vi "Correlation.vi"(9 "Y":dbl[](array[numeric]), 10 "X":dbl[](array[numeric])) -> (2 "c":dbl)   [LabVIEW 2013]
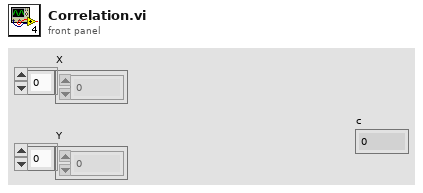
[diagram p1: front panel]
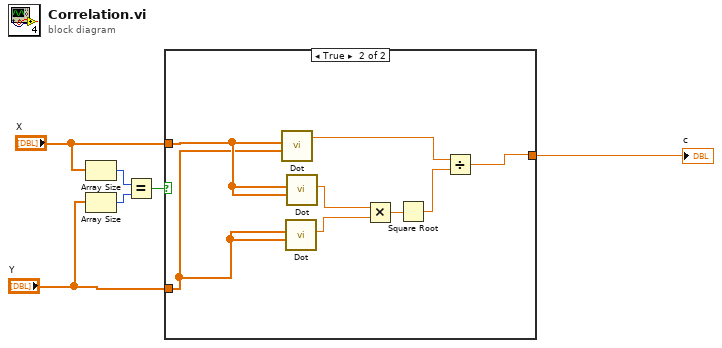
[diagram p0: block diagram]
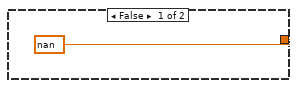
[diagram p2: hidden frame]
diagram:
  n1 = Array Size(array="X") -> (size(s)=w4:i32)
  n2 = Array Size(array="Y") -> (size(s)=w2:i32)
  n3 = Equal?(x=w4, y=w2) -> (x = y?=w5:bool)
  n4 = case shown="True" w5 {
    tunnel: "X" -> [_ w13]
    tunnel: [nan w15] -> w6
    tunnel: "Y" -> [_ w12]
    frame False {
    }
    frame True {
      n5 = call "Dot.vi"("Points Ajustés"=w12, "Y"=w13) -> ("dot(X,Y)"=w14:dbl)  [unwired: 9 in]
      n6 = call "Dot.vi"("Points Ajustés"=w12, "Y"=w12) -> ("dot(X,Y)"=w10:dbl)  [unwired: 9 in]
      n7 = call "Dot.vi"("Points Ajustés"=w13, "Y"=w13) -> ("dot(X,Y)"=w11:dbl)  [unwired: 9 in]
      n8 = Multiply(x=w11, y=w10) -> (x*y=w9:dbl)
      n9 = Square Root(x=w9) -> (sqrt(x)=w8:dbl)
      n10 = Divide(x=w14, y=w8) -> (x/y=w15:dbl)
    }
  }
  "c" <- w6
